vi "Clear Warnings.vi"(8 "error in":errorcluster, 11 "Fault Handler in":refnum<class "Fault Handler.lvclass">) -> (0 "error out":errorcluster, 3 "Fault Handler out":refnum<class "Fault Handler.lvclass">)   [LabVIEW 2023, in "Fault Handler.lvlib" / "Fault Handler.lvclass"]
doc: "Clear all warnings in the active warnings record, then it will call <b>Refresh Display</b>"
uses:
  Library/Fault Handler.lvclass
  Library/Fault Handler.lvclass/Fault Handler.ctl
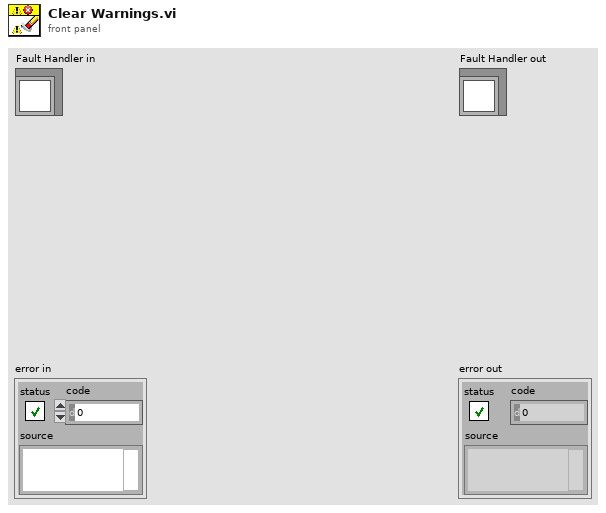
[diagram p1: front panel]
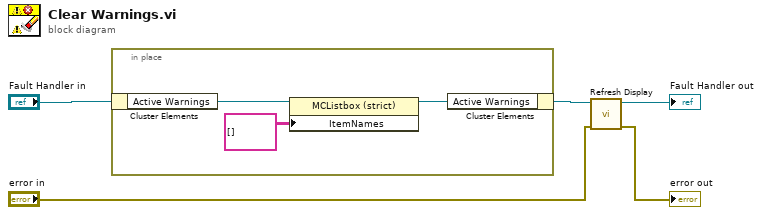
[diagram p0: block diagram]
diagram:
  n1 = in-place {
    n2 = in-place-cluster #1("Fault Handler in") -> ("Active Warnings"=w7:refnum<vi>)
    n3 = property class="MCListbox (strict)"(reference=w7, "ItemNames"=string[][] [] ("Item Names")) -> (reference out=w6:refnum<vi>)  [unwired: 1 in, 1 out]
    n4 = in-place-cluster #1("Active Warnings"=w6) -> (w1:refnum<class "Fault Handler.lvclass">)
  }
  n5 = call "Refresh Display.vi"("error in"="error in", "Fault Handler in"=w1) -> ("error out"=→"error out":errorcluster, "Fault Handler out"=→"Fault Handler out":refnum<class "Fault Handler.lvclass">)  [unwired: 8 in]
